vi "Init PowerSupply.vi"(8 "error in (no error)":errorcluster, 11 "PowerSupply-Fix in":refnum<class "PowerSupply-Fix.lvclass">) -> (0 "error out":errorcluster, 3 "PowerSupply-Fix out":refnum<class "PowerSupply-Fix.lvclass">)   [LabVIEW 2020, in "LAF2024Q2.lvlib" / "PowerSupply-Fix.lvclass"]
uses:
  PowerSupply-Fix.lvclass
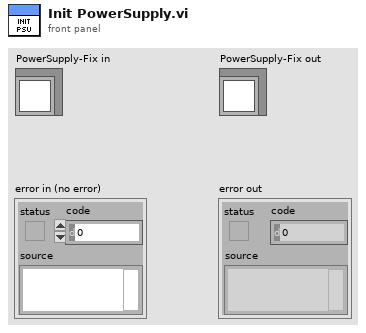
[diagram p1: front panel]
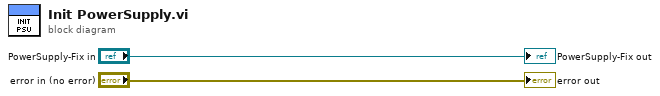
[diagram p0: block diagram]
diagram:
  "error out" <- "error in (no error)"
  "PowerSupply-Fix out" <- "PowerSupply-Fix in"
